vi "Hall Effect Animator.vi"(4 "Animation Settings":T1={"Number of Particles"=10, "px/s"=250, "Origin"={"X"=300, "Y"=150}, "Jitter"=1.0, "Seperation"=40, "X Max"=410}, 5 "Reset":bool, 11 "Gravity":dbl(slide)=0.0059880239520958695 scale=-1.0..1.0) -> (1 "Particles":cluster{"X":i32, "Y":i32}[](array[cluster]), 3 "new picture":picture)   [LabVIEW 2014]
uses:
  <vilib>/picture/picture.llb/imagedata.ctl
panel:
  in  "Pict Ring":u16(ring)
  out "Array":i32[](array[numeric])
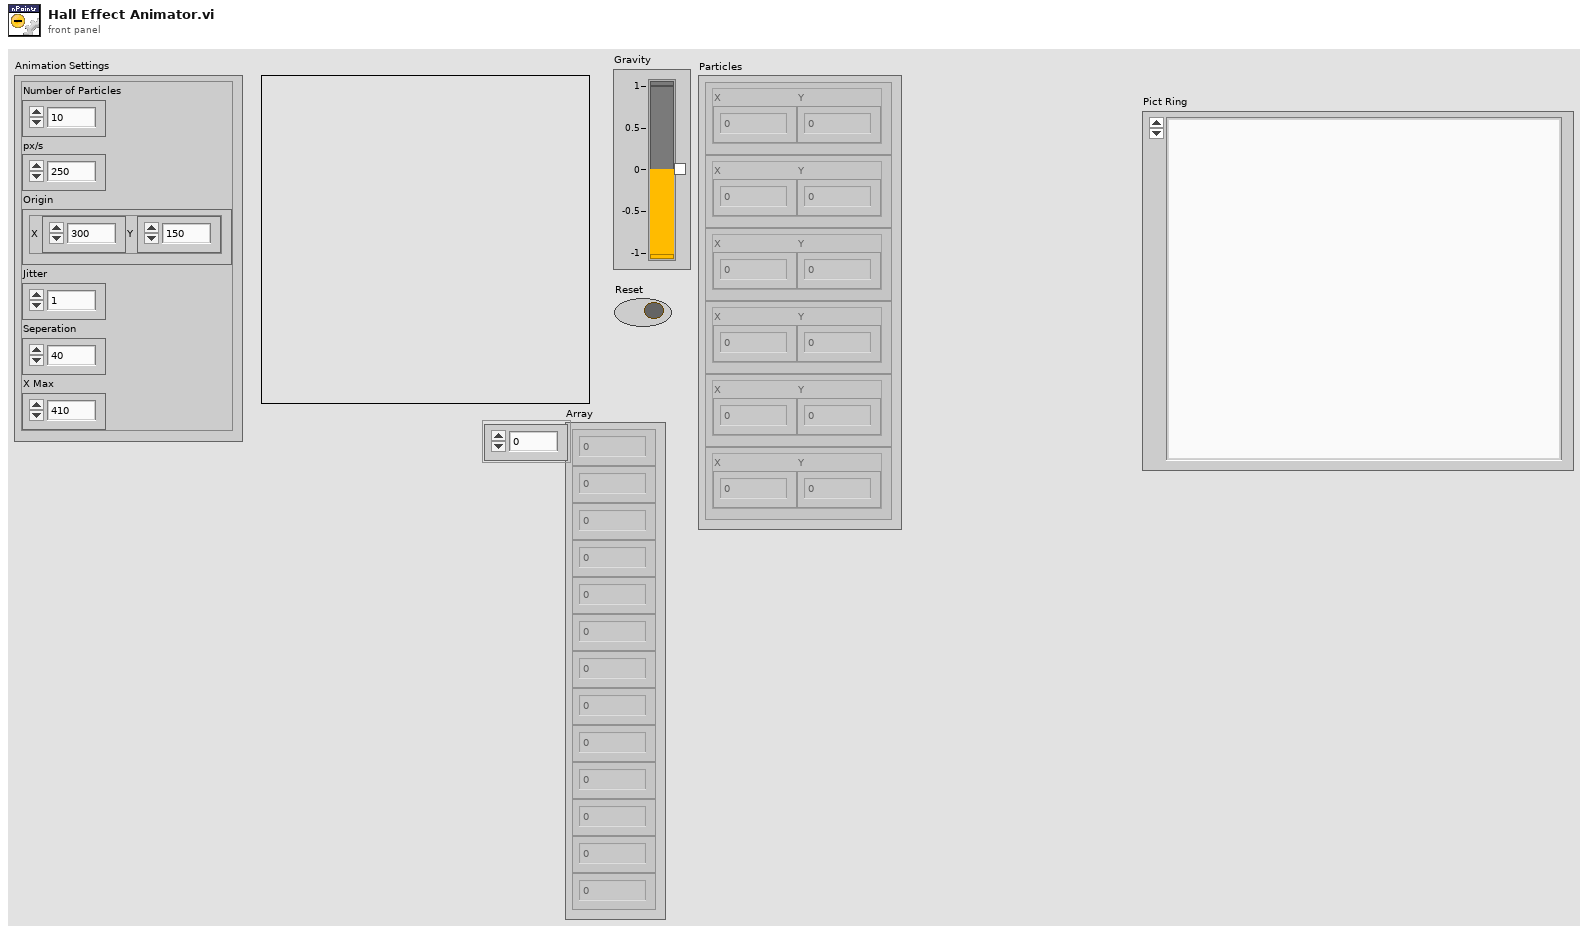
[diagram p1: front panel]
types:
  T1 = cluster{"Number of Particles":u32, "px/s":i32, "Origin":cluster{"X":i32, "Y":i32}, "Jitter":dbl, "Seperation":i32, "X Max":i32}
  T2 = typedef "imagedata.ctl" = cluster{"image type":i32, "image depth":i32, "image":u8[], "mask":u8[], "colors":u32[], "Rectangle":cluster{"left":i16, "top":i16, "right":i16, "bottom":i16}}
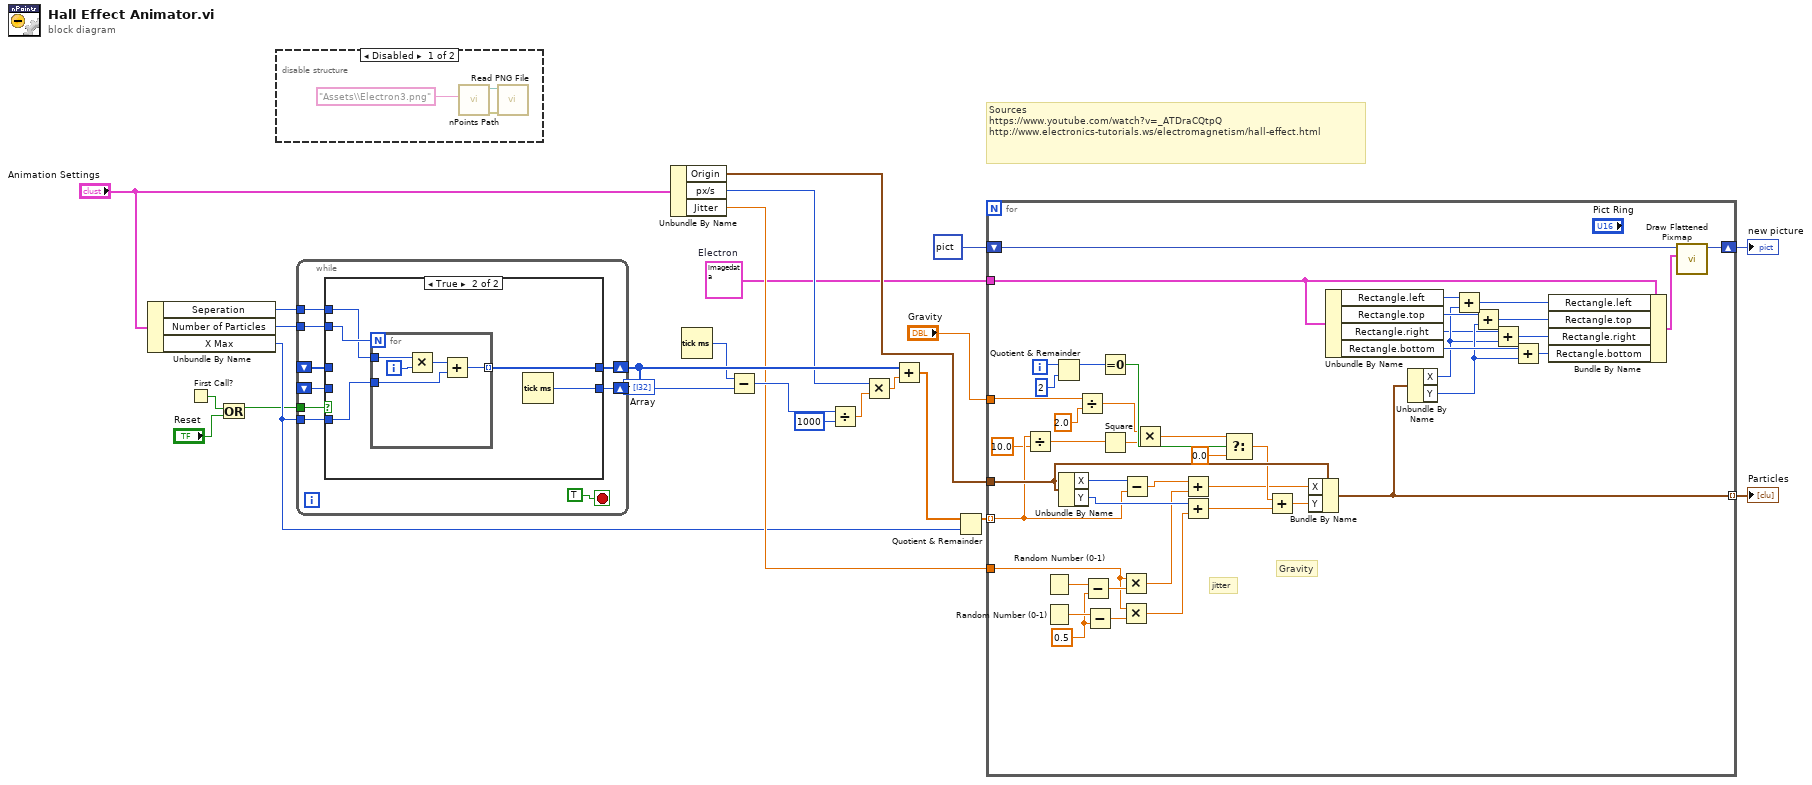
[diagram p0: block diagram]
diagram:
  w1 = T2 {"image type"=0, "image depth"=32, "image"=array[3136 elements], "mask"=[0, 63, 224, 0, 1, 255, 248, 0, 3, 255, 252, 0, 15, 255, 255, 0, 31, 255, 255, 128, 31, 255, 255, 128, 63, 255, 255, 192, 127, 255, 255, 224, 127, 255, 255, 224, 255, 255, 255, 224, 255, 255, 255, 240, 255, 255, 255, 240, 255, 255, 255, 240, 255, 255, 255, 240, 255, 255, 255, 240, 255, 255, 255, 240, 255, 255, 255, 240, 255, 255, 255, 240, 127, 255, 255, 240, 127, 255, 255, 224, 127, 255, 255, 224, 63, 255, 255, 192, 31, 255, 255, 128, 31, 255, 255, 128, 15, 255, 255, 0, 3, 255, 252, 0, 1, 255, 248, 0, 0, 127, 192, 0], "colors"=[], "Rectangle"={"left"=0, "top"=0, "right"=28, "bottom"=28}}  # Electron
  # "Sources\nhttps://www.youtube.com/watch?v=_ATDraCQtpQ\nhttp://www.electronics-tutorials.ws/electromagnetism/hall-effect.html"
  n1 = Unbundle By Name("Animation Settings") -> ("Seperation"=w9:i32, "Number of Particles"=w10:u32, "X Max"=w5:i32)
  n2 = First Call?() -> (First Call?: T/F=w22:bool)
  n3 = Or(x=w22, y="Reset") -> (x .or. y?=w4:bool)
  n4 = disable-structure shown="Disabled" {
    frame Disabled {
      n5 = call "nPoints Path.vi"("name or relative path"="Assets\\Electron3.png") -> ("error out"=w27:errorcluster, "File path"=w26:path)  [unwired: 9 in]
      n6 = call <vilib>:"Read PNG File.vi"("error in (no error)"=w27, "path to PNG file"=w26) -> ()  [unwired: 7 in, 3 out]
    }
    frame Enabled {
    }
  }
  n7 = while {
    tunnel: w4 -> [w34]
    tunnel: w5 -> [w33]
    shift-right: [w35] -> w23
    shift-left: _ -> [w31]
    shift-right: [w36] -> w24
    shift-left: _ -> [w30]
    tunnel: w10 -> [w29]
    tunnel: w9 -> [w28]
    stop <- TRUE stop-if-true
    n8 = case shown="True" w34 {
      tunnel: [w37 w43] -> w36
      tunnel: [w38 w42] -> w35
      tunnel: w33 -> [_ w41]
      tunnel: w31 -> [w38 _]
      tunnel: w30 -> [w37 _]
      tunnel: w29 -> [_ w40]
      tunnel: w28 -> [_ w39]
      frame False {
      }
      frame True {
        n9 = for {
          N: w40 -> [_]
          tunnel: [w46] -> w43 mode=indexing
          tunnel: w41 -> [w45]
          tunnel: w39 -> [w44]
          i -> [w47]
          n10 = Multiply(x=w44, y=w47) -> (x*y=w48:i32)
          n11 = Add(x=w48, y=w45) -> (x+y=w46:i32)
        }
        n12 = Tick Count (ms)() -> (millisecond timer value=w42:u32)
      }
    }
  }
  "Array" <- w24
  n13 = Unbundle By Name("Animation Settings") -> ("Origin"=w2:cluster{"X":i32, "Y":i32}, "px/s"=w7:i32, "Jitter"=w6:dbl)
  n14 = Tick Count (ms)() -> (millisecond timer value=w17:u32)
  n15 = Subtract(x=w17, y=w23) -> (x-y=w16:u32)
  n16 = Divide(x=w16, y=u32 1000) -> (x/y=w14:dbl)
  n17 = Multiply(x=w7, y=w14) -> (x*y=w13:dbl)
  n18 = Add(x=w24, y=w13) -> (x+y=w19:dbl[])
  n19 = Quotient & Remainder(x=w19, y=w5) -> (x-y*floor(x/y)=w12:dbl[])  [unwired: 1 out]
  n20 = for {
    shift-right: [w92] -> w21
    shift-left: picture data[5B] ("new picture") -> [w91]
    tunnel: w12 -> [w53] mode=indexing
    tunnel: w2 -> [w89]
    tunnel: w1 -> [w78]
    tunnel: [w76] -> w18 mode=indexing
    tunnel: "Gravity" -> [w51]
    tunnel: w6 -> [w50]
    i -> [w58]
    w73 = 0.5 ("Rand Scale")
    # "Gravity"
    # "jitter"
    n21 = Divide(x=w53, y=10.0 ("x")) -> (x/y=w54:dbl)
    n22 = Random Number (0-1)() -> (number: 0 to 1=w75:dbl)
    n23 = Random Number (0-1)() -> (number: 0 to 1=w74:dbl)
    n24 = Quotient & Remainder(x=w58, y=2) -> (x-y*floor(x/y)=w67:i32)  [unwired: 1 out]
    n25 = Unbundle By Name(w89) -> ("X"=w90:i32, "Y"=w70:i32)
    n26 = Divide(x=w51, y=2.0 ("x")) -> (x/y=w57:dbl)
    n27 = Subtract(x=w75, y=w73) -> (x-y=w72:dbl)
    n28 = Subtract(x=w74, y=w73) -> (x-y=w71:dbl)
    n29 = Equal To 0?(x=w67) -> (x = 0?=w65:bool)
    n30 = Square(x=w54) -> (x^2=w55:dbl)
    n31 = Multiply(x=w50, y=w72) -> (x*y=w69:dbl)
    n32 = Multiply(x=w50, y=w71) -> (x*y=w68:dbl)
    n33 = Subtract(x=w90, y=w53) -> (x-y=w66:dbl)
    n34 = Multiply(x=w57, y=w55) -> (x*y=w64:dbl)
    n35 = Add(x=w66, y=w69) -> (x+y=w61:dbl)
    n36 = Add(x=w70, y=w68) -> (x+y=w60:dbl)
    n37 = Select(t=w64, s=w65, f=0.0) -> (s? t:f=w62:dbl)
    n38 = Add(x=w62, y=w60) -> (x+y=w59:dbl)
    n39 = Bundle By Name(cluster=w89, "X"=w61, "Y"=w59) -> (w76:cluster{"X":i32, "Y":i32})
    n40 = Unbundle By Name(w78) -> ("Rectangle.left"=w79:i16, "Rectangle.top"=w85:i16, "Rectangle.right"=w81:i16, "Rectangle.bottom"=w87:i16)
    n41 = Unbundle By Name(w76) -> ("X"=w82:i32, "Y"=w84:i32)
    n42 = Add(x=w79, y=w82) -> (x+y=w80:i32)
    n43 = Add(x=w85, y=w84) -> (x+y=w86:i32)
    n44 = Add(x=w81, y=w82) -> (x+y=w83:i32)
    n45 = Add(x=w87, y=w84) -> (x+y=w88:i32)
    n46 = Bundle By Name(cluster=w78, "Rectangle.left"=w80, "Rectangle.top"=w86, "Rectangle.right"=w83, "Rectangle.bottom"=w88) -> (w77:T2)
    n47 = call <vilib>:"Draw Flattened Pixmap.vi"("image data"=w77, "picture"=w91) -> ("new picture"=w92:picture)  [unwired: 7 in]
  }
  "new picture" <- w21
  "Particles" <- w18
